vi "DAQ_DECM Initialize.vi"(0 "Input Terminal":tag="/CoreDIO/PFI0", 5 "Counter - Edge Counting":tag="CoreDIO/ctr0", 7 "Counter - Timer":tag="CoreDIO/ctr1", 11 "error in":errorcluster) -> (4 "DAQmx Tasks":T1, 15 "error out":errorcluster)   [LabVIEW 2021, in "DAQ_Digital Edge Count Measurement.lvlib"]
doc: "Initialize Counter task and Timer task for digital edge count measurement task.\n\nTwo tasks are used for Digital Edge Count Measurement. <B>Counter task</B> is used for edge counting and <B>Timer task</B> is used to control precise measurement window for edge counting by generating a single pulse of required measurement time and it is used for <B>hardware timed wait type</B>. This generated pulse will be internally used by Counter task. No external physical connections are required. \n\nNOTE: Leave <B>Counter - Timer</B> input empty for <B>software timed wait type</B>.\n\nRefer detailed help for more details on hardware timed vs software timed wait types."
uses:
  DAQ_Digital Edge Count Measurement.lvlib
  Typedefs/DAQmx Tasks.ctl
  <vilib>/DAQmx/create/channels.llb/DAQmx Create Channel (CI-Count Edges).vi
  <vilib>/DAQmx/create/channels.llb/DAQmx Create Channel (CO-Pulse Generation-Time).vi
  <resource>/objmgr/daqmx.rc
panel:
  # "Inputs"
  # "Outputs"
  # "Overview:\nThis VI initializes the counter input channel for digital edge count measurement task and provides the DAQmx Task Out\n\nHardware Requirement: A compatible PXI, PCIe, USB, cDAQ or Testscale device\n\nSoftware Requirement: NI DAQmx 2022Q4 or later\n\nInstructions:\n1. Enter input terminal where digital events should be counted in Input Terminal.\n2. Enter a counter resources for Counter task which is used for edge counting.\n3. Enter a counter resources for Timer task which is used to generate measurement window. Skip this input for software timed operations. Refer detailed help of this VI for more details on hardware timed vs software timed digital edge counting.\n4. Get both Counter and Timer tasks from DAQmx Tasks.\n\nNotes: \n1. User can use the DAQmx Tasks on other VI in this library to configure and initiate count digital events task.\n2. Two tasks are used for Digital Events Count Measurement. Counter task is used for edge counting and Timer task is used to control precise measurement window for edge counting by generating a single pulse of required measurement time and it is used for hardware timed wait type."
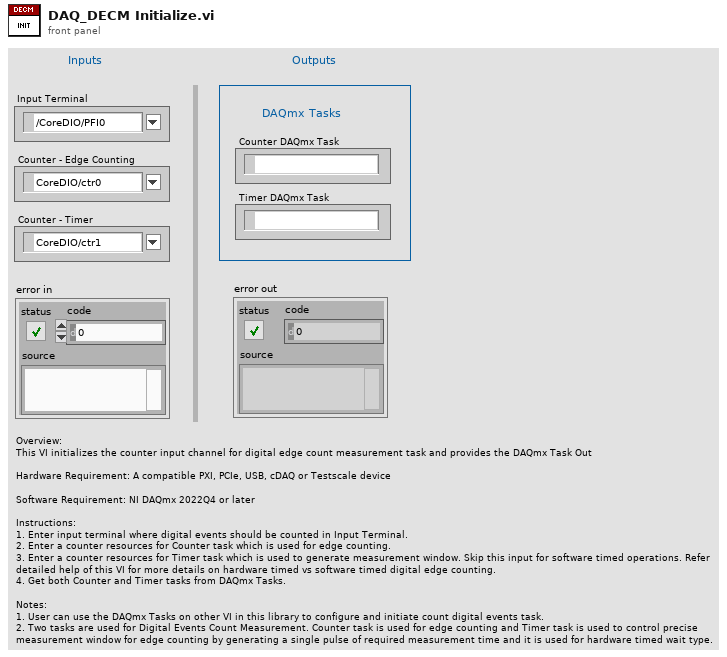
[diagram p1: front panel]
types:
  T1 = typedef "DAQ_Digital Edge Count Measurement.lvlib/DAQmx Tasks.ctl" = cluster{"Counter DAQmx Task":refnum<k21>, "Timer DAQmx Task":refnum<k21>}
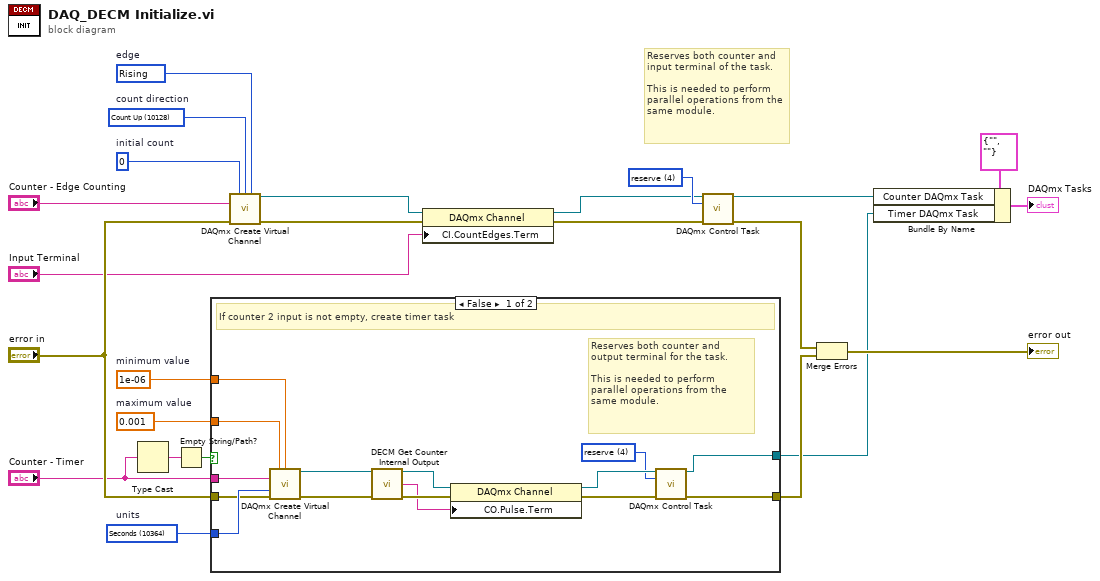
[diagram p0: block diagram]
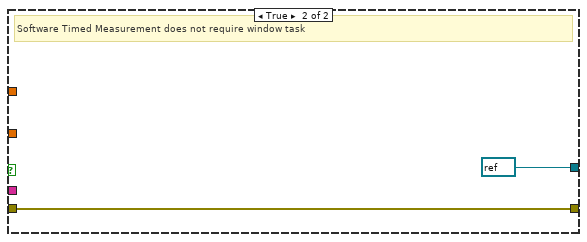
[diagram p2: hidden frame]
diagram:
  w13 = 1e-06  # minimum value
  w14 = 0.001  # maximum value
  w15 = 10364 items=["Seconds"=10364]  # units
  w16 = u32 0  # initial count
  w17 = 10280 items=["Rising"=10280, "Falling"=10171]  # edge
  w18 = 10128 items=["Count Up"=10128, "Count Down"=10124, "Externally Controlled"=10326]  # count direction
  w24 = 4 items=["verify"=2, "reserve"=4, "commit"=3, "unreserve"=5, "abort"=6] ("action")
  # "Reserves both counter and input terminal of the task.\n\nThis is needed to perform parallel operations from the same module."
  n1 = Type Cast(x="Counter - Timer") -> (*(type *) &x=w8:string)  [unwired: 1 in]
  n2 = Empty String/Path?(string/path=w8) -> (empty?=w9:bool)
  n3 = case shown="False" w9 {
    tunnel: [w37 refnum<k21> refnum ("task out")] -> w4
    tunnel: w15 -> [w35 _]
    tunnel: w14 -> [w34 _]
    tunnel: w13 -> [w33 _]
    tunnel: "error in" -> [w32 w41]
    tunnel: [w31 w41] -> w10
    tunnel: "Counter - Timer" -> [w30 _]
    frame False {
      w36 = 4 items=["verify"=2, "reserve"=4, "commit"=3, "unreserve"=5, "abort"=6] ("action")
      # "Reserves both counter and output terminal for the task.\n\nThis is needed to perform parallel operations from the same module."
      # "If counter 2 input is not empty, create timer task"
      n4 = call-poly <vilib>:"DAQmx Create Virtual Channel.vi"("high time"=w34, "low time"=w33, "counter"=w30, "units"=w35, "error in"=w32) -> ("task out"=w29:refnum<k21>, "error out"=w28:errorcluster)  [unwired: 9 in]
      n5 = call "DECM Get Counter Internal Output.vi"("DAQmx Task In"=w29, "error in"=w28) -> ("DAQmx Task Out"=w27:refnum<k21>, "Internal Counter Output"=w25:tag, "error out"=w26:errorcluster)  [unwired: 11 in]
      n6 = property class="DAQmx Channel"(reference=w27, error in=w26, "CO.Pulse.Term"=w25) -> (reference out=w39:refnum<k21>, error out=w38:errorcluster)
      n7 = call <vilib>:"DAQmx Control Task.vi"("task/channels in"=w39, "action"=w36, "error in"=w38) -> ("task out"=w37:refnum<k21>, "error out"=w31:errorcluster)  [unwired: 11 in]
    }
    frame True {
      # "Software Timed Measurement does not require window task"
    }
  }
  n8 = call-poly <vilib>:"DAQmx Create Virtual Channel.vi"("initial count"=w16, "count direction"=w18, "edge"=w17, "counter"="Counter - Edge Counting", "error in"="error in") -> ("task out"=w20:refnum<k21>, "error out"=w22:errorcluster)  [unwired: 9 in]
  n9 = property class="DAQmx Channel"(reference=w20, error in=w22, "CI.CountEdges.Term"="Input Terminal") -> (reference out=w19:refnum<k21>, error out=w21:errorcluster)
  n10 = call <vilib>:"DAQmx Control Task.vi"("task/channels in"=w19, "action"=w24, "error in"=w21) -> ("task out"=w5:refnum<k21>, "error out"=w23:errorcluster)  [unwired: 11 in]
  n11 = Merge Errors(w23, w10) -> (→"error out":errorcluster)
  n12 = Bundle By Name(cluster=T1 {"Counter DAQmx Task"="", "Timer DAQmx Task"=""} ("DAQmx Tasks"), "Counter DAQmx Task"=w5, "Timer DAQmx Task"=w4) -> (→"DAQmx Tasks":T1)
